vi "Temperature Limitgyy.vi"() -> ()   [LabVIEW 2013]
doc: "该VI可仿真温度采集，绘制温度图形，并通知用户温度是否超出范围。"
panel:
  in  "开始":bool
  in  "△t(ms)":i32(slide)=400 scale=50.0..500.0
  in  "停止":bool
  in  "上限":dbl=28.0 format="%.2f"
  out "温度":cluster{"Temperature":dbl, "High Limit":dbl}(graph)={"Temperature"=85.88749999999999, "High Limit"=80.0}
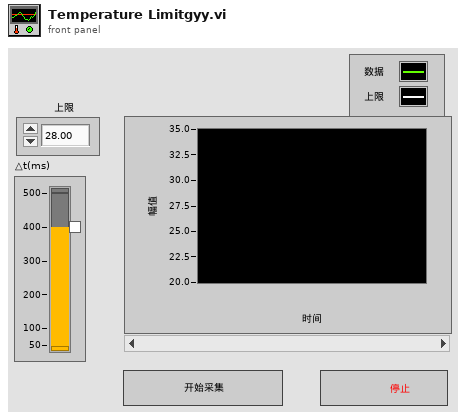
[diagram p1: front panel]
types:
  T1 = enum16{"Always On", "Always Off", "Off While Running"}
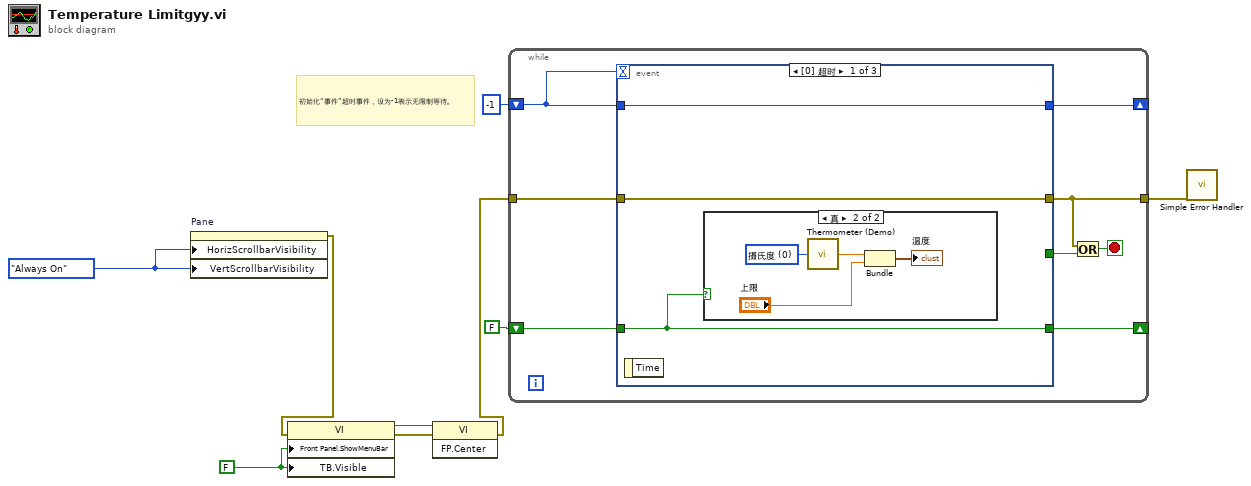
[diagram p0: block diagram]
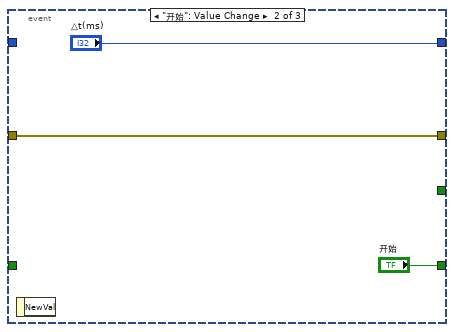
[diagram p3: hidden frame]
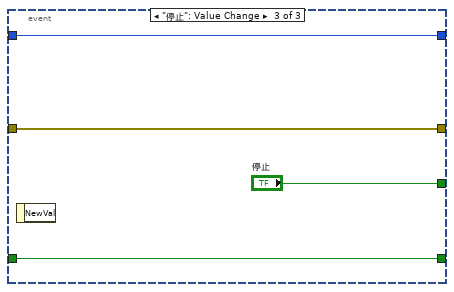
[diagram p4: hidden frame]
diagram:
  w5 = FALSE ("工具栏:可见")
  w6 = T1."Always On" ("水平滚动条可见")
  # "初始化“事件”超时事件，设为-1表示无限制等待。"
  n1 = property on="Pane" class="Pane"("HorizScrollbarVisibility"=w6, "VertScrollbarVisibility"=w6) -> (error out=w2:errorcluster)  [unwired: 2 in, 1 out]
  n2 = property on="属性节点" class="VI"(error in=w2, "Front Panel.ShowMenuBar"=w5, "TB.Visible"=w5) -> (reference out=w4:refnum<vi>, error out=w3:errorcluster)  [unwired: 1 in]
  n3 = invoke on="调用节点" class="VI" method="FP.Center"(reference=w4, error in=w3) -> (error out=w1:errorcluster)  [unwired: 1 in, 2 out]
  n4 = while {
    tunnel: w1 -> [w17]
    tunnel: [w15] -> w8
    shift-right: [w13] -> _
    shift-left: FALSE ("开始") -> [w12]
    shift-right: [w11] -> _
    shift-left: -1 ("△t(ms)") -> [w10]
    stop <- w16 stop-if-true
    n5 = event shown="[0] 超时" {
      selector: _ -> [_ _ _]
      dyn-events: _ -> [_ _ _]
      timeout: w10 -> [_ _ _]
      tunnel: [_ _ "停止"] -> w14
      tunnel: w17 -> [w20 w25 w30]
      tunnel: [w20 w25 w30] -> w15
      tunnel: [w18 "开始" w29] -> w13
      tunnel: w12 -> [w18 _ w29]
      tunnel: [w19 "△t(ms)" w28] -> w11
      tunnel: w10 -> [w19 _ w28]
      event Timeout {
        n6 = event-data ("事件数据节点")() -> ()  [unwired: 1 in, 1 out]
        n7 = case shown="真" w18 {
          frame False {
          }
          frame True {
            w21 = u16 0 items=["摄氏度", "华氏度"] ("单位（0：摄氏度）")
            n8 = call "Thermometer (Demo).vi"("单位（0：摄氏度）"=w21) -> ("温度值"=w22:dbl)
            n9 = Bundle ("捆绑")("温度值"=w22, "上限"="上限") -> (→"温度":cluster{"温度值":dbl, "上限":dbl})  [unwired: 1 in]
          }
        }
      }
      event "开始": Value Change {
        n10 = event-data ("事件数据节点")() -> ()  [unwired: 1 in, 1 out]
      }
      event "停止": Value Change {
        n11 = event-data ("事件数据节点")() -> ()  [unwired: 1 in, 1 out]
      }
    }
    n12 = Or ("或")(x=w15, y=w14) -> (x .or. y?=w16:bool)
  }
  n13 = call <vilib>:"Simple Error Handler.vi"("error in (no error)"=w8) -> ()  [unwired: 4 in, 5 out]
